vi "Write IInstrument Base.vi"(8 "error in (no error)":errorcluster, 10 "IInstrument Base":refnum<class "IInstrument.lvclass">, 11 "IVirtual Instrument in":refnum<class "IVirtual Instrument.lvclass">) -> (0 "error out":errorcluster, 3 "IVirtual Instrument out":refnum<class "IVirtual Instrument.lvclass">)   [LabVIEW 2023, in "IVirtual Instrument.lvclass"]
uses:
  IVirtual Instrument.lvclass
  IInstrument/IInstrument.lvclass
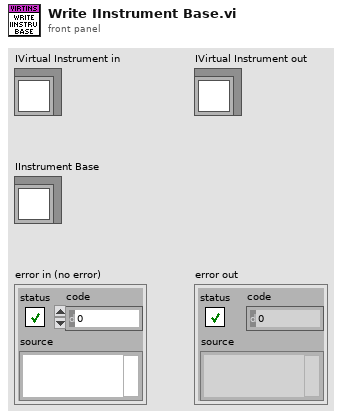
[diagram p1: front panel]
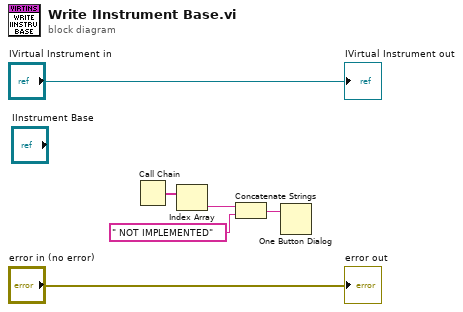
[diagram p0: block diagram]
diagram:
  n1 = Call Chain() -> (call chain=w4:string[])
  n2 = Index Array(array=w4) -> (element=w1:string)  [unwired: 1 in]
  n3 = Concatenate Strings(w1, " NOT IMPLEMENTED" ("string")) -> (w3:string)
  n4 = One Button Dialog(message=w3) -> ()  [unwired: 1 in, 1 out]
  "error out" <- "error in (no error)"
  "IVirtual Instrument out" <- "IVirtual Instrument in"
